vi "sample2String.vi"(1 "Precision (1-6)":i16, 2 "Number":dbl format="%#_13g", 3 "Label":string) -> (0 "Output String":string)   [LabVIEW 2017]
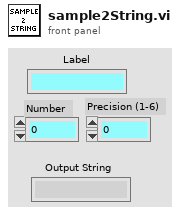
[diagram p1: front panel]
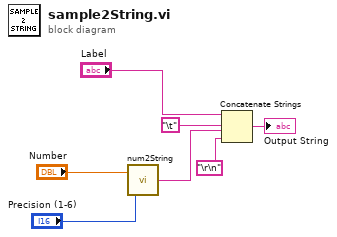
[diagram p0: block diagram]
diagram:
  n1 = call "num2String.vi"("Precision (1-6)"="Precision (1-6)", "Number"="Number") -> ("F-format String"=w5:string)
  n2 = Concatenate Strings("Label", "\t", w5, "\r\n") -> (→"Output String":string)
